vi "SubVI_Button.vi"(11 "VI 입력":refnum<vi>) -> (2 "Button":i32, 3 "Exit Button":bool)   [LabVIEW 2023]
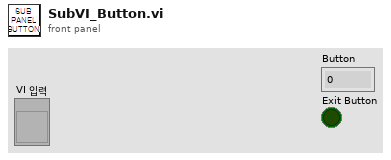
[diagram p1: front panel]
types:
  T1 = enum32{"선택 없음", "Select 1", "Select 2", "Select 3", "Select 4"}
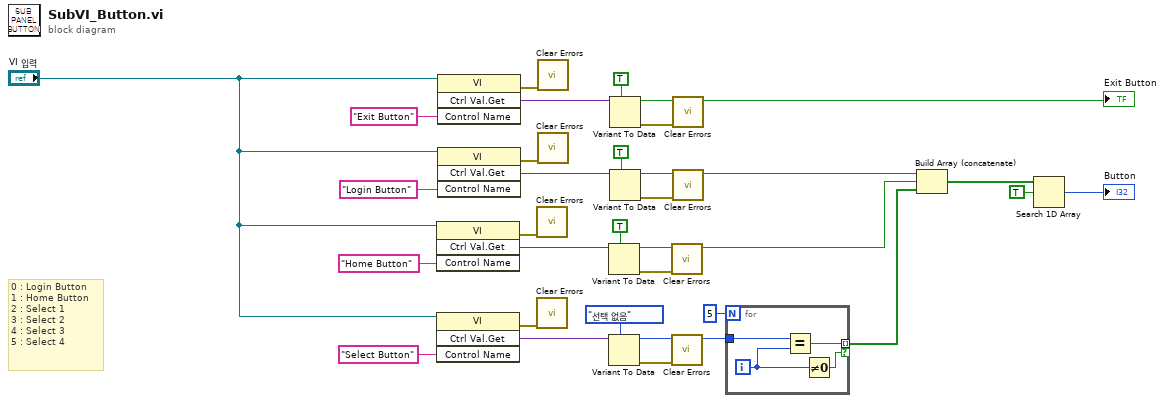
[diagram p0: block diagram]
diagram:
  # "0 : Login Button\n1 : Home Button\n2 : Select 1\n3 : Select 2\n4 : Select 3\n5 : Select 4"
  n1 = invoke class="VI" method="Ctrl Val.Get"(reference="VI 입력", "Control Name"="Home Button" ("컨트롤 이름")) -> (error out=w26:errorcluster, "Get Control Value Variant"=w27:variant)  [unwired: 2 in, 2 out]
  n2 = invoke class="VI" method="Ctrl Val.Get"(reference="VI 입력", "Control Name"="Select Button" ("컨트롤 이름")) -> (error out=w16:errorcluster, "Get Control Value Variant"=w24:variant)  [unwired: 2 in, 2 out]
  n3 = invoke class="VI" method="Ctrl Val.Get"(reference="VI 입력", "Control Name"="Exit Button" ("컨트롤 이름")) -> (error out=w5:errorcluster, "Get Control Value Variant"=w6:variant)  [unwired: 2 in, 2 out]
  n4 = invoke class="VI" method="Ctrl Val.Get"(reference="VI 입력", "Control Name"="Login Button" ("컨트롤 이름")) -> (error out=w20:errorcluster, "Get Control Value Variant"=w21:variant)  [unwired: 2 in, 2 out]
  n5 = call <vilib>:"Clear Errors.vi"("error in (no error)"=w26) -> ()  [unwired: 5 in, 2 out]
  n6 = call <vilib>:"Clear Errors.vi"("error in (no error)"=w16) -> ()  [unwired: 5 in, 2 out]
  n7 = call <vilib>:"Clear Errors.vi"("error in (no error)"=w5) -> ()  [unwired: 5 in, 2 out]
  n8 = call <vilib>:"Clear Errors.vi"("error in (no error)"=w20) -> ()  [unwired: 5 in, 2 out]
  n9 = Variant To Data(type=TRUE ("Auto Dispose Reference"), Variant=w27) -> (data=w8:bool, error out=w29:errorcluster)  [unwired: 1 in]
  n10 = Variant To Data(type=T1."선택 없음" ("Select Button"), Variant=w24) -> (data=w17:T1, error out=w15:errorcluster)  [unwired: 1 in]
  n11 = Variant To Data(type=TRUE ("Auto Dispose Reference"), Variant=w6) -> (data=→"Exit Button":bool, error out=w3:errorcluster)  [unwired: 1 in]
  n12 = Variant To Data(type=TRUE ("Auto Dispose Reference"), Variant=w21) -> (data=w9:bool, error out=w18:errorcluster)  [unwired: 1 in]
  n13 = call <vilib>:"Clear Errors.vi"("error in (no error)"=w29) -> ()  [unwired: 5 in, 2 out]
  n14 = call <vilib>:"Clear Errors.vi"("error in (no error)"=w15) -> ()  [unwired: 5 in, 2 out]
  n15 = call <vilib>:"Clear Errors.vi"("error in (no error)"=w3) -> ()  [unwired: 5 in, 2 out]
  n16 = call <vilib>:"Clear Errors.vi"("error in (no error)"=w18) -> ()  [unwired: 5 in, 2 out]
  n17 = for {
    N: 5 -> [_]
    tunnel: w17 -> [w34]
    tunnel: [w33] -> w14 mode=indexing if=w31
    i -> [w32]
    n18 = Equal?(x=w34, y=w32) -> (x = y?=w33:bool)
    n19 = Not Equal To 0?(x=w32) -> (x != 0?=w31:bool)
  }
  n20 = Build Array (concatenate)(w9, w8, w14) -> (w12:bool[])
  n21 = Search 1D Array(1D array=w12, element=TRUE ("원소")) -> (index of element=→"Button":i32)  [unwired: 1 in]
